vi "DIO IRQ 4-bit.vi"(4 "IRQ NO":u8[](array[numeric]), 6 "IRQ CNT":u32[](array[numeric]), 7 "FIFO In":refnum<k21>="DIO A IRQ", 8 "IRQ.FALL":fxp<+,4,4> format="%08b", 9 "IRQ.RISE":fxp<+,4,4> format="%08b", 10 "IRQ.ENA":fxp<+,4,4> format="%08b", 11 "IN 3:0":fxp<+,4,4>) -> ()   [LabVIEW 2021]
uses:
  <vilib>/rvi/Emulation/niFpgaSctlEmulationGetInTimedLoop.vi
  <vilib>/Utility/error.llb/Clear Errors.vi
  <vilib>/rvi/DataTransferAndStorage/Container/Common/niFpgaContainerExecOnDevCompGetState.vi
  <vilib>/rvi/Emulation/niFpgaEmulationIsFPGAContextNoSignature.vi
  <vilib>/rvi/errors/niFpgaSetErrorForExecOnDevCompSimple.vi
  <vilib>/rvi/eio/common/nirviEmuReportErrorAndStop.vi
  <vilib>/rvi/DataTransferAndStorage/Container/Common/niFpgaContainerGetUniqueNameForEmu.vi
  <vilib>/rvi/FIFO/Fifo_Resource/nirvififoEmulationSetSize.vi
  <vilib>/rvi/FIFO/Fifo_Resource/nirviFifoEmulationQueueMgr.vi
  <instcachedir>/0/nirviFifoEmulationQueueMgr_E5CAEC123FF24DC58D834DCA3CDAA9B5.lvgen/nirviFifoEmulationQueueMgr_E5CAEC123FF24DC58D834DCA3CDAA9B5_005.vi
  <vilib>/rvi/FIFO/Fifo_Resource/nirvififoEmulationDetermineInputValidOut.vi
  <vilib>/rvi/FIFO/Fifo_Resource/nirvififoEmulationCreateLock.vi
  <vilib>/rvi/Emulation/niFpgaProcessEmulError.vi
  <vilib>/rvi/FIFO/Fifo_Resource/nirvififoEmulationObtainLock.vi
  <vilib>/rvi/FIFO/Fifo_Resource/nirvififoEmulationReleaseLock.vi
  <vilib>/rvi/occurrence/nirviWaitOnOccurrenceBase.vi
  <vilib>/rvi/errors/nirviReportUnexpectedCaseInternalError.vi
  <vilib>/rvi/errors/nirviReportUnexpectedCaseInternalError (U32).vi
  <vilib>/rvi/interface/RandomDataEmulation/niFpgaRandomDataHandleErrors.vi
  <vilib>/rvi/DataTransferAndStorage/Container/XNode/niFpgaContainer.xnode
  <vilib>/rvi/FIFO/Fifo_Resource/niFpgaFifoEmulationRefIn.vi
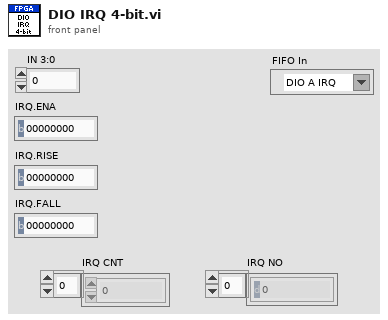
[diagram p1: front panel]
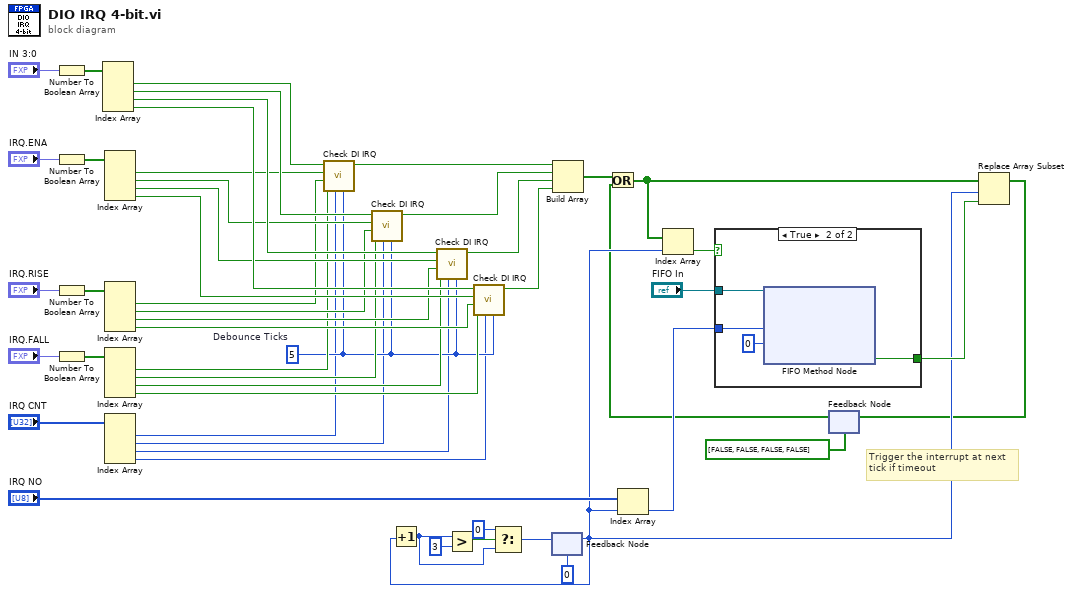
[diagram p0: block diagram]
diagram:
  w27 = u16 5  # Debounce Ticks
  # "Trigger the interrupt at next \ntick if timeout"
  n1 = Number To Boolean Array(number="IN 3:0") -> (Boolean array=w45:bool[])
  n2 = Number To Boolean Array(number="IRQ.ENA") -> (Boolean array=w50:bool[])
  n3 = Number To Boolean Array(number="IRQ.RISE") -> (Boolean array=w48:bool[])
  n4 = Number To Boolean Array(number="IRQ.FALL") -> (Boolean array=w46:bool[])
  n5 = Index Array(array=w45) -> (element #1=w43:bool, element #2=w42:bool, element #3=w41:bool, element #4=w40:bool)  [unwired: 4 in]
  n6 = Index Array(array=w50) -> (element #1=w39:bool, element #2=w38:bool, element #3=w37:bool, element #4=w36:bool)  [unwired: 4 in]
  n7 = Index Array(array=w48) -> (element #1=w35:bool, element #2=w34:bool, element #3=w33:bool, element #4=w32:bool)  [unwired: 4 in]
  n8 = Index Array(array=w46) -> (element #1=w31:bool, element #2=w30:bool, element #3=w29:bool, element #4=w28:bool)  [unwired: 4 in]
  n9 = Index Array(array="IRQ CNT") -> (element #1=w25:u32, element #2=w24:u32, element #3=w23:u32, element #4=w22:u32)  [unwired: 4 in]
  n10 = call "Check DI IRQ.vi"("Debounce Ticks"=w27, "Count"=w25, "On Falling Edge?"=w31, "On Rising Edge?"=w35, "Enable Interrupt?"=w39, "Digital In"=w43) -> ("Trigger?"=w21:bool)  [unwired: 5 in]
  n11 = call "Check DI IRQ.vi"("Debounce Ticks"=w27, "Count"=w24, "On Falling Edge?"=w30, "On Rising Edge?"=w34, "Enable Interrupt?"=w38, "Digital In"=w42) -> ("Trigger?"=w20:bool)  [unwired: 5 in]
  n12 = call "Check DI IRQ.vi"("Debounce Ticks"=w27, "Count"=w23, "On Falling Edge?"=w29, "On Rising Edge?"=w33, "Enable Interrupt?"=w37, "Digital In"=w41) -> ("Trigger?"=w19:bool)  [unwired: 5 in]
  n13 = call "Check DI IRQ.vi"("Debounce Ticks"=w27, "Count"=w22, "On Falling Edge?"=w28, "On Rising Edge?"=w32, "Enable Interrupt?"=w36, "Digital In"=w40) -> ("Trigger?"=w18:bool)  [unwired: 5 in]
  n14 = feedback #1(u8 0) -> (w9:u8)
  n15 = Increment(x=w9) -> (x+1=w5:u8)
  n16 = Greater?(x=w5, y=u8 3) -> (0:w7:bool)
  n17 = Select(t=u8 0, s=w7, f=w5) -> (s? t:f=w4:u8)
  n18 = feedback-in #1(w4) -> ()
  n19 = Build Array(w21, w20, w19, w18) -> (w14:bool[])
  n20 = Index Array(array="IRQ NO", index=w9) -> (element=w15:u8)
  n21 = feedback #2(bool[] [FALSE, FALSE, FALSE, FALSE] ("initialized array")) -> (w1:bool[])
  n22 = Or(x=w14, y=w1) -> (x .or. y?=w11:bool[])
  n23 = Index Array(array=w11, index=w9) -> (element=w13:bool)
  n24 = case shown="True" w13 {
    selector: w13 -> [w52 _]
    tunnel: [w52 w54] -> w12
    tunnel: w15 -> [_ w55]
    tunnel: "FIFO In" -> [_ w53]
    frame False {
    }
    frame True {
      n25 = xnode ("FIFO Method Node")("Element"=w55, "Timeout"=0, "FIFO In"=w53) -> ("Timed Out?"=w54:bool)  [unwired: 1 out]
    }
  }
  n26 = Replace Array Subset(array=w11, new element=w12, index=w9) -> (w2:bool[])
  n27 = feedback-in #2(w2) -> ()
